vi "NI VeriStand - Print Debug Line.vi"(7 "Attribute":T1=7 items=["Plain White"=7, "Bold White"=15, "Bold Blue"=9, "Bold Green"=10, "Bold Red"=12], 8 "error in (no error)":errorcluster, 9 "Append newline? (T)":bool=TRUE, 10 "Add to log file? (F)":bool, 11 "Message":string) -> (0 "error out":errorcluster)   [LabVIEW 2020, in "Custom Device Utility Library.lvlib"]
uses:
  <vilib>/NI VeriStand/Custom Device Tools/Custom Device Utility Library/Custom Device Utility Library.lvlib
  <vilib>/NI VeriStand/Custom Device Tools/Custom Device Utility Library/RT Debug String Color Spec.ctl
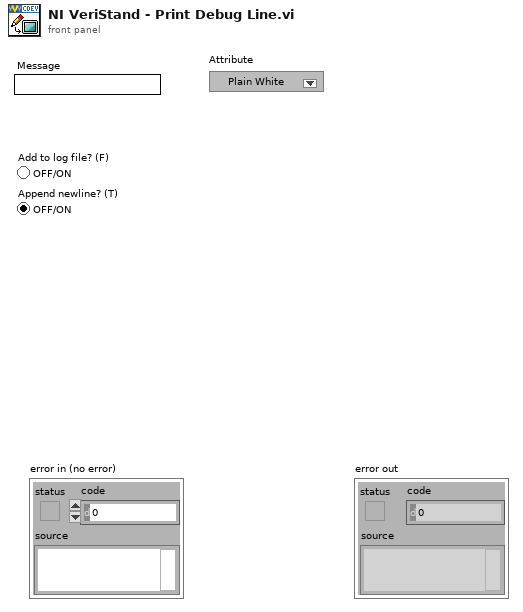
[diagram p1: front panel]
types:
  T1 = typedef "Custom Device Utility Library.lvlib/RT Debug String Color Spec.ctl" = u16
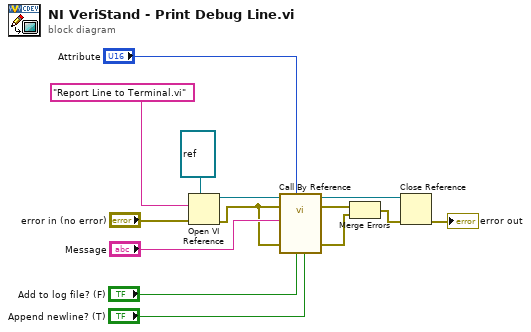
[diagram p0: block diagram]
diagram:
  n1 = Open VI Reference(type specifier VI Refnum (for type only)=refnum<vi> refnum, vi path="Report Line to Terminal.vi", error in (no error)="error in (no error)") -> (vi reference=w11:refnum<vi>, error out=w9:errorcluster)  [unwired: 3 out]
  n2 = call-by-ref "?"(reference=w11, error in=w9, "Append newline? (T)"="Append newline? (T)", "Add to log file? (T)"="Add to log file? (F)", "Color (Plain White)"="Attribute", 8:"error in (no error)"=w9, "Message"="Message") -> (reference out=w4:refnum<vi>, error out=w8:errorcluster, 0:"error out"=w7:errorcluster)  [unwired: 6 in]
  n3 = Merge Errors(w8, w7) -> (w3:errorcluster)
  n4 = Close Reference(reference=w4, error in (no error)=w3) -> (error out=→"error out":errorcluster)
